vi "CRYSet Login setup Front Panel.vi"(11 "Vi Ref in":refnum<vi> caption="Vi Ref") -> (3 "Vi Ref out":refnum<vi> caption="Vi Ref")   [LabVIEW 2013]
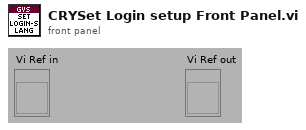
[diagram p1: front panel]
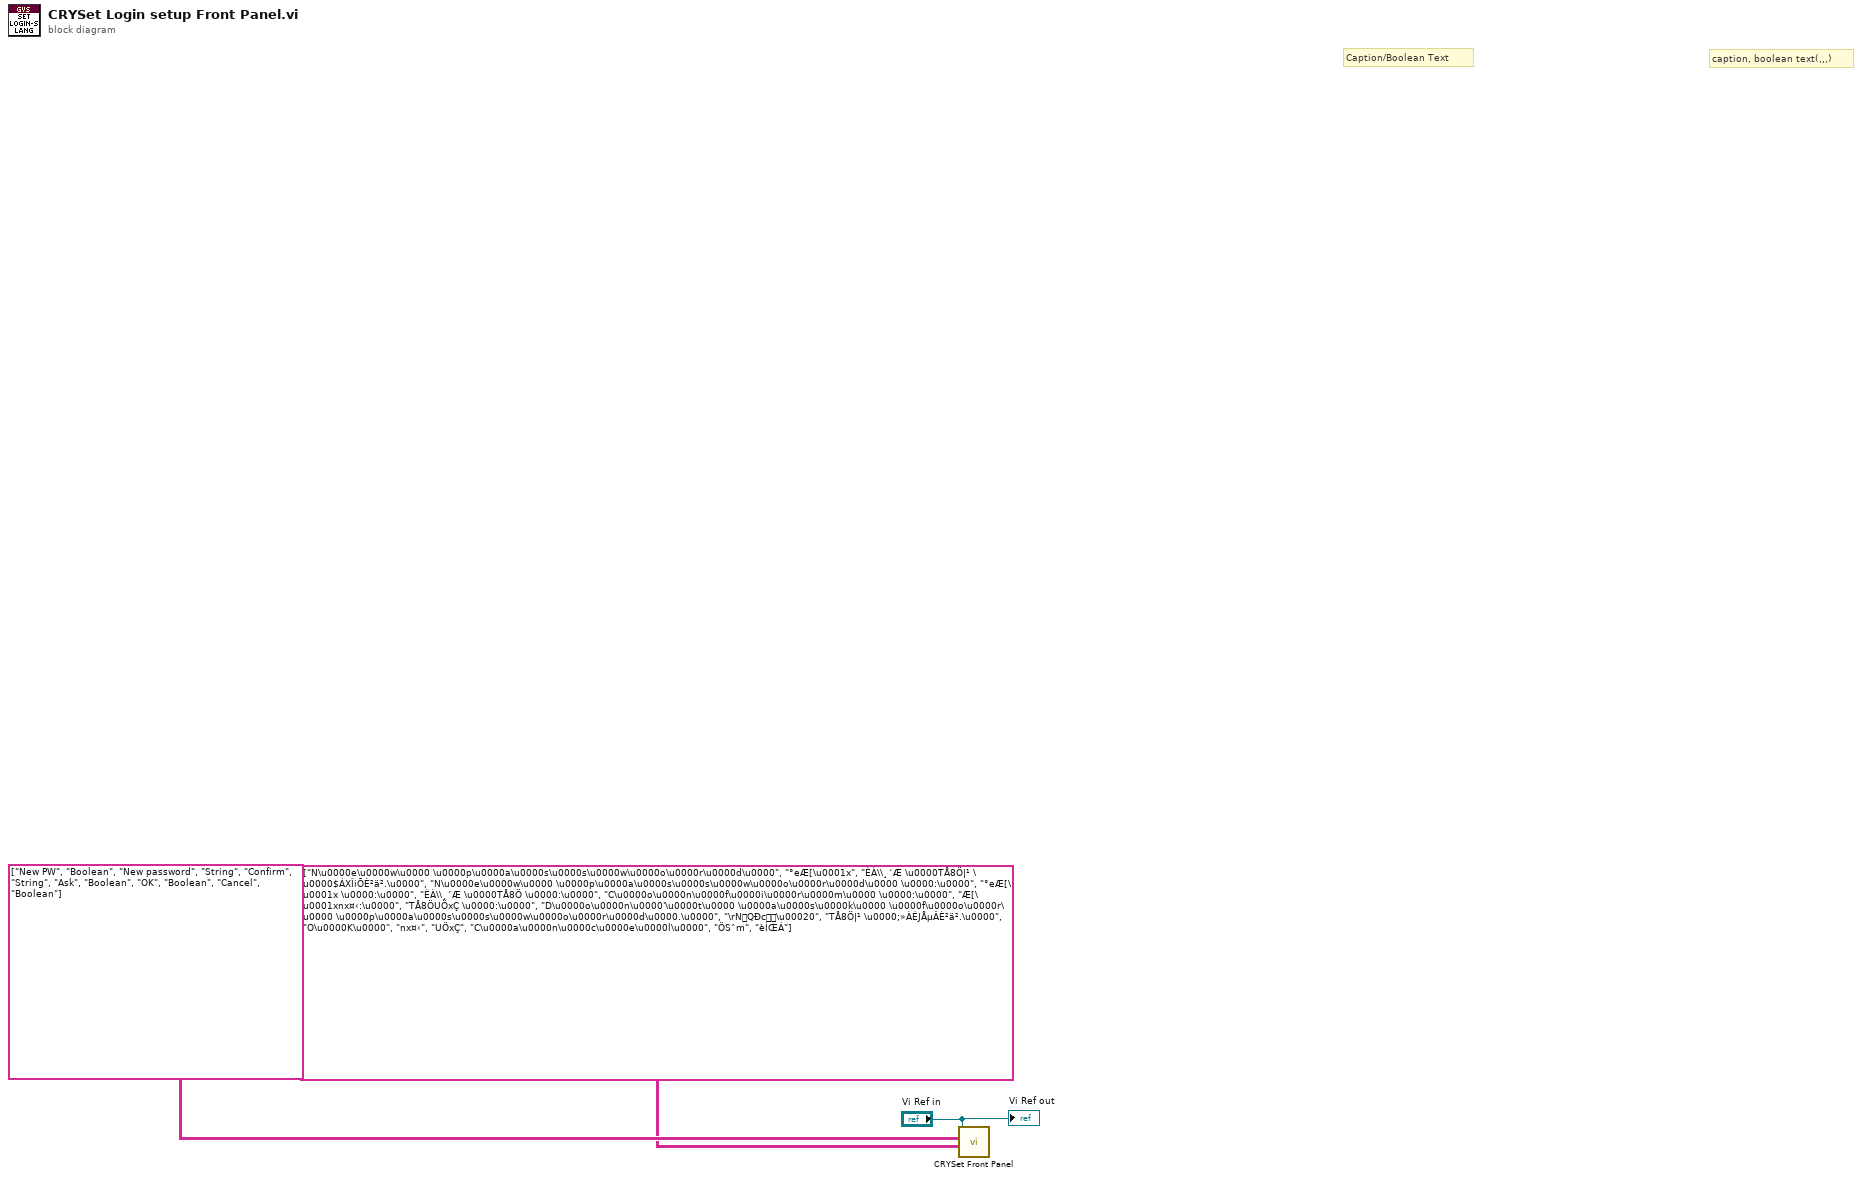
[diagram p0: block diagram]
diagram:
  # "caption, boolean text(,,,)"
  # "Caption/Boolean Text"
  n1 = call "CRYSet Front Panel.vi"("Caption(Boolean Text)"=string[][] [["N\u0000e\u0000w\u0000 \u0000p\u0000a\u0000s\u0000s\u0000w\u0000o\u0000r\u0000d\u0000", "°eÆ[\u0001x", "ÈÀ\\¸´Æ \u0000TÅ8Ö|¹ \u0000$ÁXÎiÕÈ²ä².\u0000"], ["N\u0000e\u0000w\u0000 \u0000p\u0000a\u0000s\u0000s\u0000w\u0000o\u0000r\u0000d\u0000 \u0000:\u0000", "°eÆ[\u0001x \u0000:\u0000", "ÈÀ\\¸´Æ \u0000TÅ8Ö \u0000:\u0000"], ["C\u0000o\u0000n\u0000f\u0000i\u0000r\u0000m\u0000 \u0000:\u0000", "Æ[\u0001xnx¤‹:\u0000", "TÅ8ÖUÖxÇ \u0000:\u0000"], ["D\u0000o\u0000n\u0000'\u0000t\u0000 \u0000a\u0000s\u0000k\u0000 \u0000f\u0000o\u0000r\u0000 \u0000p\u0000a\u0000s\u0000s\u0000w\u0000o\u0000r\u0000d\u0000.\u0000", "\rNQÐc\u00020", "TÅ8Ö|¹ \u0000;»ÀÉJÅµÂÈ²ä².\u0000"], ["O\u0000K\u0000", "nx¤‹", "UÖxÇ"], ["C\u0000a\u0000n\u0000c\u0000e\u0000l\u0000", "ÖSˆm", "èÍŒÁ"]], "Control ID and Type(Label Name, Type)"=string[][] [["New PW", "Boolean"], ["New password", "String"], ["Confirm", "String"], ["Ask", "Boolean"], ["OK", "Boolean"], ["Cancel", "Boolean"]], "Vi Ref"="Vi Ref in") -> ()  [unwired: 9 in]
  "Vi Ref out" <- "Vi Ref in"
